vi "WLC.vi"(3 "output control":T1, 4 "data":T2, 5 "F (pN)":dbl[](array[numeric])=[0.0, 0.047244094488188976, 0.09448818897637795, 0.14173228346456693, 0.1889763779527559, 0.23622047244094488, 0.28346456692913385, 0.33070866141732286, 0.3779527559055118, 0.4251968503937008, 0.47244094488188976, 0.5196850393700787, 0.5669291338582677, 0.6141732283464567, 0.6614173228346457, 0.7086614173228346, 0.7559055118110236, 0.8031496062992126, 0.8503937007874016, 0.8976377952755905, 0.9448818897637795, 0.9921259842519685, 1.0393700787401574, 1.0866141732283465, 1.1338582677165354, 1.1811023622047243, 1.2283464566929134, 1.2755905511811023, 1.3228346456692914, 1.3700787401574803, 1.4173228346456692, 1.4645669291338583, 1.5118110236220472, 1.5590551181102361, 1.6062992125984252, 1.6535433070866141, 1.7007874015748032, 1.7480314960629921, 1.795275590551181, 1.8425196850393701, 1.889763779527559, 1.937007874015748, 1.984251968503937, 2.031496062992126, 2.078740157480315, 2.125984251968504, 2.173228346456693, 2.220472440944882, 2.267716535433071, 2.3149606299212597, 2.3622047244094486, 2.409448818897638, 2.456692913385827, 2.5039370078740157, 2.5511811023622046, 2.5984251968503935, 2.645669291338583, 2.6929133858267718, 2.7401574803149606, 2.7874015748031495, 2.8346456692913384, 2.8818897637795278, 2.9291338582677167, 2.9763779527559056, 3.0236220472440944, 3.0708661417322833, 3.1181102362204722, 3.1653543307086616, 3.2125984251968505, 3.2598425196850394, 3.3070866141732282, 3.354330708661417, 3.4015748031496065, 3.4488188976377954, 3.4960629921259843, 3.543307086614173, 3.590551181102362, 3.6377952755905514, 3.6850393700787403, 3.732283464566929, 3.779527559055118, 3.826771653543307, 3.874015748031496, 3.921259842519685, 3.968503937007874, 4.015748031496063, 4.062992125984252, 4.110236220472441, 4.15748031496063, 4.2047244094488185, 4.251968503937008, 4.299212598425197, 4.346456692913386, 4.393700787401575, 4.440944881889764, 4.488188976377953, 4.535433070866142, 4.582677165354331, 4.6299212598425195, 4.677165354330708, 4.724409448818897, 4.771653543307087, 4.818897637795276, 4.866141732283465, 4.913385826771654, 4.960629921259843, 5.0078740157480315, 5.05511811023622, 5.102362204724409, 5.149606299212598, 5.196850393700787, 5.244094488188976, 5.291338582677166, 5.338582677165355, 5.3858267716535435, 5.433070866141732, 5.480314960629921, 5.52755905511811, 5.574803149606299, 5.622047244094488, 5.669291338582677, 5.716535433070866, 5.7637795275590555, 5.811023622047244, 5.858267716535433, 5.905511811023622, 5.952755905511811, 6.0], 6 "a (variable only)":dbl[](array[numeric])) -> (0 "error out":errorcluster, 1 "f'(X,a)":dbl[][](array[numeric]), 2 "z (um)":dbl[](array[numeric]))   [LabVIEW 2018]
doc: "This template is the starting point for creating a model function to be passed to the Nonlinear Curve Fit.vi."
uses:
  <vilib>/gmath/NumericalOptimization/objective function data.ctl
  <vilib>/gmath/NumericalOptimization/LM_output select.ctl
  <vilib>/gmath/NI_Gmath.lvlib
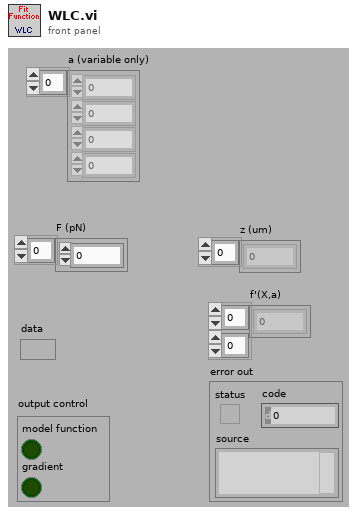
[diagram p1: front panel]
types:
  T1 = typedef "NI_Gmath.lvlib/LM_output select.ctl" = cluster{"model function":bool, "gradient":bool}
  T2 = typedef "NI_Gmath.lvlib/objective function data.ctl" = variant
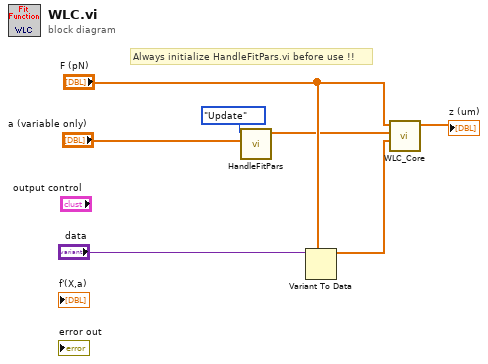
[diagram p0: block diagram]
diagram:
  # "Always initialize HandleFitPars.vi before use !!"
  n1 = call "HandleFitPars.vi"("Var params in"="a (variable only)", "Task"=enum16{"Init", "Update", "Get"}."Update") -> ("All params out"=w1:dbl[])  [unwired: 3 in, 4 out]
  n2 = Variant To Data(type="F (pN)", Variant="data") -> (data=w2:dbl[])  [unwired: 1 in, 1 out]
  n3 = call "WLC_Core.vi"("t (s)"=w2, "params in (all)"=w1, "F (pN)"="F (pN)") -> ("z (um)"=→"z (um)":dbl[])  [unwired: 5 in, 3 out]
